vi "K182singleread.vi"(8 "error in":T1, 11 "VISA resource name":refnum<visa-resource-name>) -> (0 "error out":T1, 2 "Voltage":dbl, 3 "VISA resource name out":refnum<visa-resource-name>)   [LabVIEW 2015]
panel:
  out "read buffer":string
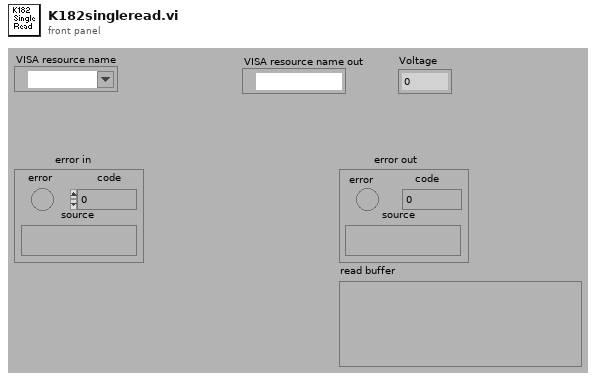
[diagram p1: front panel]
types:
  T1 = cluster{"error":bool, "code":i32, "source":string}
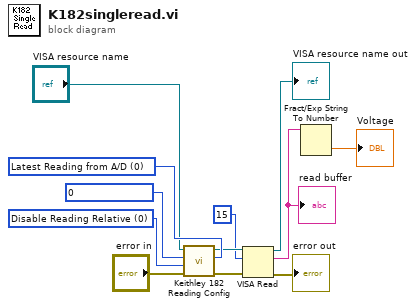
[diagram p0: block diagram]
diagram:
  w11 = u16 0 items=["Disable Reading Relative", "Enable Reading Relative using current reading", "Enable Reading Relative using Value", "Enable Reading Relative, use present value"] ("Analog Output Relative")
  w8 = u16 0 items=["Latest Reading from A/D", "One Reading from buffer", "All Readings in buffer", "Maximum Value in buffer", "Mimimum Value in buffer"] ("Reading Source")
  n1 = call "Keithley 182 Reading Config.VI"("Reading Source"=w8, "error in"="error in", "Analog Output Relative"=w11, "Reading Format"=u16 0, "VISA resource name"="VISA resource name") -> ("error out"=w5:T1, "VISA resource name out"=w3:refnum<visa-resource-name>)  [unwired: 1 in]
  n2 = VISA Read(VISA resource name=w3, byte count=u32 15, error in (no error)=w5) -> (VISA resource name out=→"VISA resource name out":refnum<visa-resource-name>, read buffer=w6:string, error out=→"error out":errorcluster)  [unwired: 1 out]
  "read buffer" <- w6
  n3 = Fract/Exp String To Number(string=w6) -> (number=→"Voltage":dbl)  [unwired: 4 out]
